vi "Read Graph Image.vi"() -> ()   [LabVIEW 2020]
uses:
  _libraries/Startup Processes/_typedefs/Subpanel Names.ctl
  <vilib>/Utility/sysdir.llb/System Directory Type.ctl
  toolbox/Standard Signalling/not_Generic Named Notifier/not_Generic Named Notifier.lvlib
  _ude/Read Graph Image/Read Graph Image.lvlib
  _libraries/Startup Processes/Startup Processes.lvlib
panel:
  out "Raw Response":variant
  out "?":picture
  out "Error Out":errorcluster
  in  "Plugin Names":T1
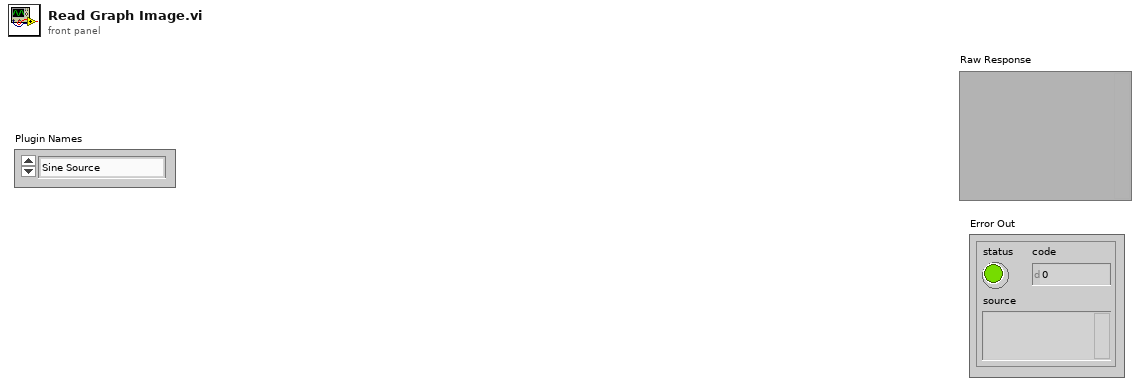
[diagram p1: front panel]
types:
  T1 = typedef "Startup Processes.lvlib/Subpanel Names.ctl" = enum16{"Sine Source", "Ramp Source", "Hen House TC", "Dog House TC", "Out House TC"}
  T2 = typedef "System Directory Type.ctl" = i32
  T3 = typedef "imagedata.ctl" = cluster{"image type":i32, "image depth":i32, "image":u8[], "mask":u8[], "colors":u32[], "Rectangle":cluster{"left":i16, "top":i16, "right":i16, "bottom":i16}}
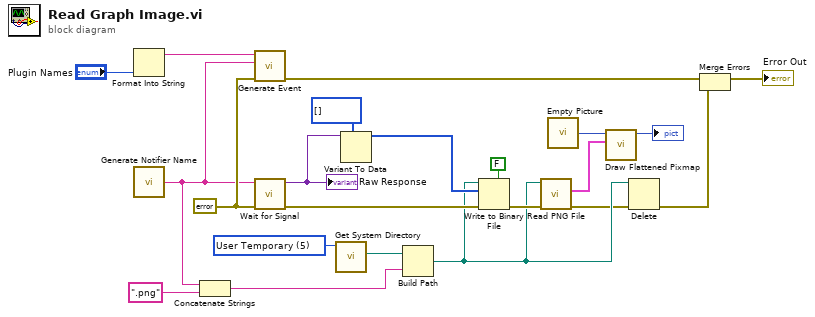
[diagram p0: block diagram]
diagram:
  w13 = T2 5 items=["User Home"=0, "User Desktop"=1, "User Documents"=2, "User Application Data"=3, "User Preferences"=4, "User Temporary"=5, "Public Documents"=6, "Public Application Data"=7, "Public Preferences"=8, "Public Cache"=13, "System Core Libraries"=9, "System Installed Libraries"=10, "Application Files"=11, "Boot Volume Root"=12] ("system directory type")
  w19 = errorcluster {"status"=FALSE, "code"=0, "source"=""} ("Error In")
  n1 = Format Into String("Plugin Names") -> (resulting string=w20:string)  [unwired: 3 in, 1 out]
  n2 = call "Generate Notifier Name.vi"() -> ("Notifier Name"=w10:string)
  n3 = Concatenate Strings(w10, ".png" ("string")) -> (w11:string)
  n4 = call "Generate Event.vi"("Error In"=w19, "Response Notifier"=w10, "Graph Name"=w20) -> ("Error Out"=w18:errorcluster)  [unwired: 4 in]
  n5 = call "Wait for Signal.vi"("Error In"=w19, "Notifier Name"=w10) -> ("Error Out"=w15:errorcluster, "Signal Data"=w1:variant)  [unwired: 4 in]
  "Raw Response" <- w1
  n6 = call <vilib>:"Get System Directory.vi"("system directory type"=w13) -> ("system directory"=w12:path)  [unwired: 10 in]
  n7 = Variant To Data(type=u8[] [] ("Waveform Graph"), Variant=w1) -> (data=w16:u8[])  [unwired: 1 in, 1 out]
  n8 = Build Path(base path=w12, name or relative path=w11) -> (appended path=w4:path)
  n9 = Write to Binary File(file (use dialog)=w4, data=w16, error in=w15, 5:FALSE ("prepend array or string size? (T)")) -> (error out=w8:errorcluster)  [unwired: 2 in, 2 out]
  n10 = call <vilib>:"Read PNG File.vi"("error in (no error)"=w8, "path to PNG file"=w4) -> ("error out"=w3:errorcluster, "image data"=w7:T3)  [unwired: 7 in, 1 out]
  n11 = call "Empty Picture"() -> ("empty picture"=w6:picture)
  n12 = call <vilib>:"Draw Flattened Pixmap.vi"("image data"=w7, "picture"=w6) -> ("new picture"=→"?":picture)  [unwired: 7 in]
  n13 = Delete(path (use dialog)=w4, error in=w3) -> (error out=w2:errorcluster)  [unwired: 3 in, 2 out]
  n14 = Merge Errors(w18, w2) -> (→"Error Out":errorcluster)
